vi "Configure Frequency.vi"(7 "Mode":enum16{"Center Span", "Start Stop"}(ring), 8 "error in (no error)":errorcluster, 9 "Span/Stop Frequency":dbl, 10 "Center/Start Frequency":dbl, 11 "VNA-FieldFox in":refnum<class "VNA-FieldFox.lvclass">) -> (0 "error out":errorcluster, 3 "VNA-FieldFox out":refnum<class "VNA-FieldFox.lvclass">)   [LabVIEW 2020, in "VNA-FieldFox.lvclass"]
doc: "Configures the frequency range for the sweep.\nThe default mode is Center Span."
uses:
  VNA-FieldFox.lvclass
  C:/Sandbox/RF Bench/Source Code/WiSpry Test Framework/Instruments/Instrument.lvclass
  Instrument.lvclass/Instrument.ctl
  Instrument.lvclass
  <instrlib>/Agilent N99XX Series/Agilent N99XX Series.lvlib
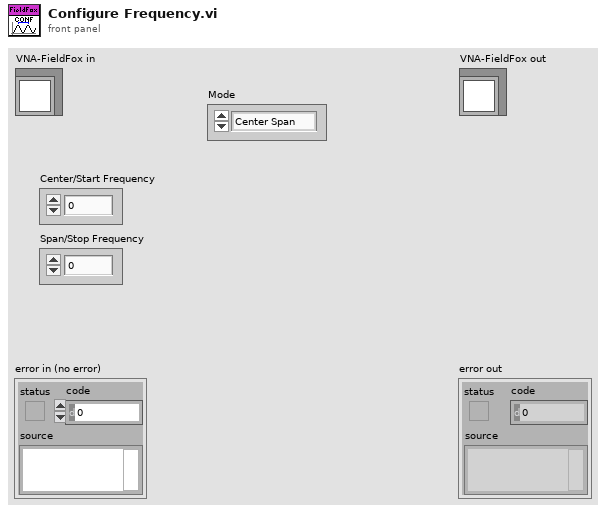
[diagram p1: front panel]
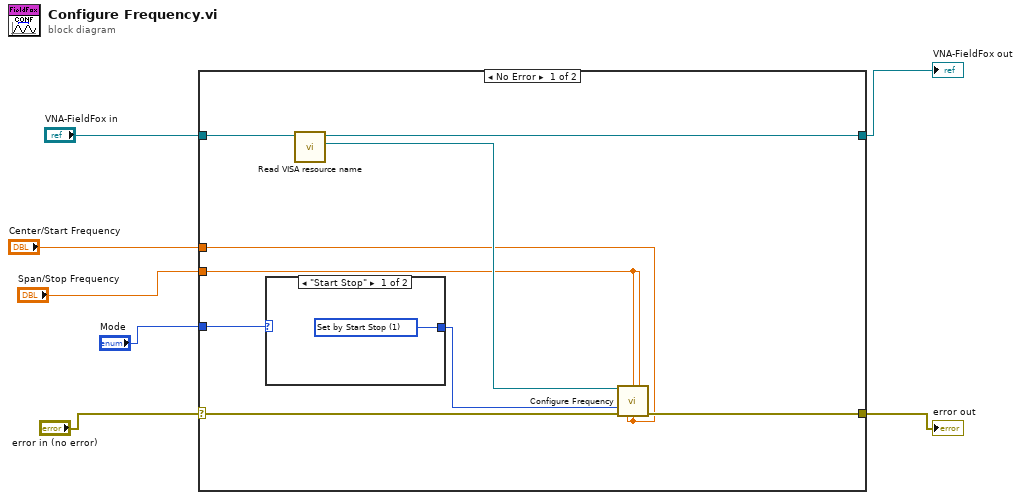
[diagram p0: block diagram]
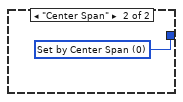
[diagram p2: hidden frame]
diagram:
  n1 = case shown="No Error" "error in (no error)" {
    selector: "error in (no error)" -> [w10 w20]
    tunnel: [w13 w20] -> w4
    tunnel: [w14 w19] -> w5
    tunnel: "VNA-FieldFox in" -> [w16 w19]
    tunnel: "Mode" -> [w15 _]
    tunnel: "Span/Stop Frequency" -> [w9 _]
    tunnel: "Center/Start Frequency" -> [w8 _]
    frame No Error {
      n2 = case shown="\"Start Stop\"" w15 {
        tunnel: [w17 w18] -> w11
        frame "Start Stop" {
          w17 = 1 items=["Set by Center Span", "Set by Start Stop"] ("Frequency Type (0: Set by Center Span)")
        }
        frame "Center Span" {
          w18 = 0 items=["Set by Center Span", "Set by Start Stop"] ("Frequency Type (0: Set by Center Span)")
        }
      }
      n3 = call "Read VISA resource name.vi"("Instrument in"=w16) -> ("VISA resource name"=w12:refnum<visa-resource-name>, "Instrument out"=w14:refnum<class "VNA-FieldFox.lvclass">)  [unwired: 9 in]
      n4 = call <instrlib>:"Configure Frequency.vi"("VISA resource name"=w12, "Span Frequency (0 Hz)"=w9, "Stop Frequency (0 Hz)"=w9, "Frequency Type (0: Set by Center Span)"=w11, "error in (no error)"=w10, "Center Frequency (2E+6 Hz)"=w8, "Start Frequency (0)"=w8) -> ("error out"=w13:errorcluster)  [unwired: 3 in, 5 out]
    }
    frame Error {
    }
  }
  "error out" <- w4
  "VNA-FieldFox out" <- w5
